vi "from_binari_data_to_variant.vi"(5 "little-endian":bool, 7 "dataType":variant, 8 "error in (no error)":errorcluster, 10 "name":string, 11 "binaryData":variant) -> (0 "error out":errorcluster, 3 "dataOut":variant)   [LabVIEW 2015, in "BSON_convertors_Library.lvlib"]
uses:
  BSON_convertors_Library.lvlib
  typedefs/binaryData_cluster.ctl
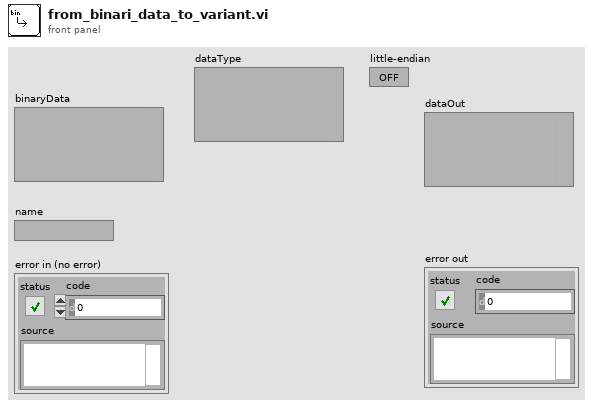
[diagram p1: front panel]
types:
  T1 = typedef "Type Descriptor Enumeration__ogtk.ctl" = enum8{"<Null>", "I8", "I16", "I32", "I64", "U8", "U16", "U32", "U64", "SGL", "DBL", "EXT", "CSG", "CDB", "CXT", "0x0F", "0x10", "0x11", "0x12", "0x13", "0x14", "Enum U8", "Enum U16", "Enum U32", "Enum U64", "SGL PQ", "DBL PQ", "EXT PQ", "CSG PQ", "CDB PQ", "CXT PQ", "0x1F", "0x20", "Boolean", "0x22", "0x23", "0x24", "0x25", "0x26", "0x27", "0x28", "0x29", "0x2A", "0x2B", "0x2C", "0x2D", "0x2E", "0x2F", "String", "0x31", "Path", "Pict", "0x34", "0x35", "0x36", "DAQ", "0x38", "0x39", "0x3A", "0x3B", "0x3C", "0x3D", "0x3E", "0x3F", "Array", "0x41", "0x42", "0x43", "0x44", "0x45", "0x46", "0x47", "0x48", "0x49", "0x4A", "0x4B", "0x4C", "0x4D", "0x4E", "0x4F", "Cluster", "0x51", "0x52", "Variant", "Waveform", "0x55", "0x56", "0x57", "0x58", "0x59", "0x5A", "0x5B", "0x5C", "0x5D", "0x5E", "0x5F", "0x60", "0x61", "0x62", "0x63", "0x64", "0x65", "0x66", "0x67", "0x68", "0x69", "0x6A", "0x6B", "0x6C", "0x6D", "0x6E", "0x6F", "Refnum"}
  T2 = typedef "BSON_convertors_Library.lvlib/binaryData_cluster.ctl" = cluster{"subType":u8, "byteArray":u8[]}
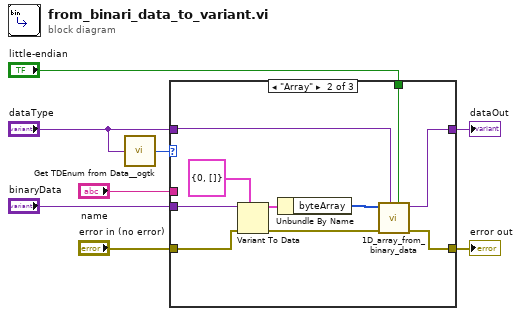
[diagram p0: block diagram]
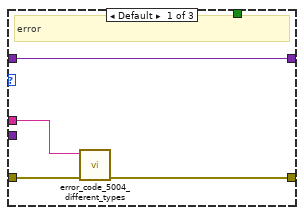
[diagram p2: hidden frame]
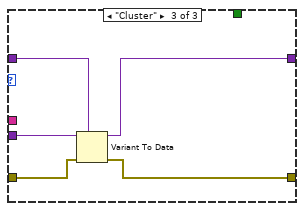
[diagram p3: hidden frame]
diagram:
  n1 = call <userlib>:"Get TDEnum from Data__ogtk.vi"("Data"="dataType") -> ("Type Descriptor Enumeration"=w1:T1)  [unwired: 4 in]
  n2 = case shown="\"Array\"" w1 {
    tunnel: "error in (no error)" -> [w11 w19 w24]
    tunnel: "binaryData" -> [_ w22 w27]
    tunnel: [w12 w14 w23] -> w4
    tunnel: "name" -> [w10 _ _]
    tunnel: "dataType" -> [w9 w16 w26]
    tunnel: [w9 w15 w25] -> w7
    tunnel: "little-endian" -> [_ w13 _]
    frame Default {
      # "error"
      n3 = call "error_code_5004_different_types.vi"("error in (no error)"=w11, "name"=w10) -> ("error out"=w12:errorcluster)  [unwired: 9 in]
    }
    frame "Array" {
      n4 = Variant To Data(error in=w19, type=T2 {"subType"=0, "byteArray"=[]} ("binaryData"), Variant=w22) -> (data=w20:T2, error out=w17:errorcluster)
      n5 = Unbundle By Name(w20) -> ("byteArray"=w18:u8[])
      n6 = call "1D_array_from_binary_data.vi"("little-endian?"=w13, "inputArray(type)"=w16, "error in (no error)"=w17, "byteArray"=w18) -> ("error out"=w14:errorcluster, "dataArray"=w15:variant)  [unwired: 6 in]
    }
    frame "Cluster" {
      n7 = Variant To Data(error in=w24, type=w26, Variant=w27) -> (data=w25:variant, error out=w23:errorcluster)
    }
  }
  "dataOut" <- w7
  "error out" <- w4
